vi "Charging_Configure.vi"(7 "file path (Rounded Square Wave Array)":path=path "C:/ATS Development/Code/Drivers/Charging/Rounded_Square_Wave_Array", 8 "error in (no error)":errorcluster, 10 "waveform settings":T1={"Frequency (40000 Hz)"=40000.0, "Offset (0 V)"=0.0, "Gain (3.7)"=3.7}, 11 "logical name (\"SampleFGen\")":refnum<k15> caption="instrument handle") -> (0 "error out":errorcluster, 1 "Arbitrary Waveform Handle [ARB]":i32, 3 "instrument handle out":refnum<k15>)   [LabVIEW 2010]
uses:
  <vilib>/Utility/file.llb/Read From Spreadsheet File (DBL).vi
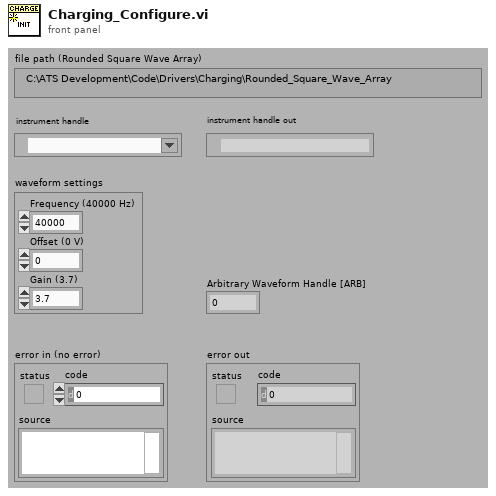
[diagram p1: front panel]
types:
  T1 = cluster{"Frequency (40000 Hz)":dbl, "Offset (0 V)":dbl, "Gain (3.7)":dbl}
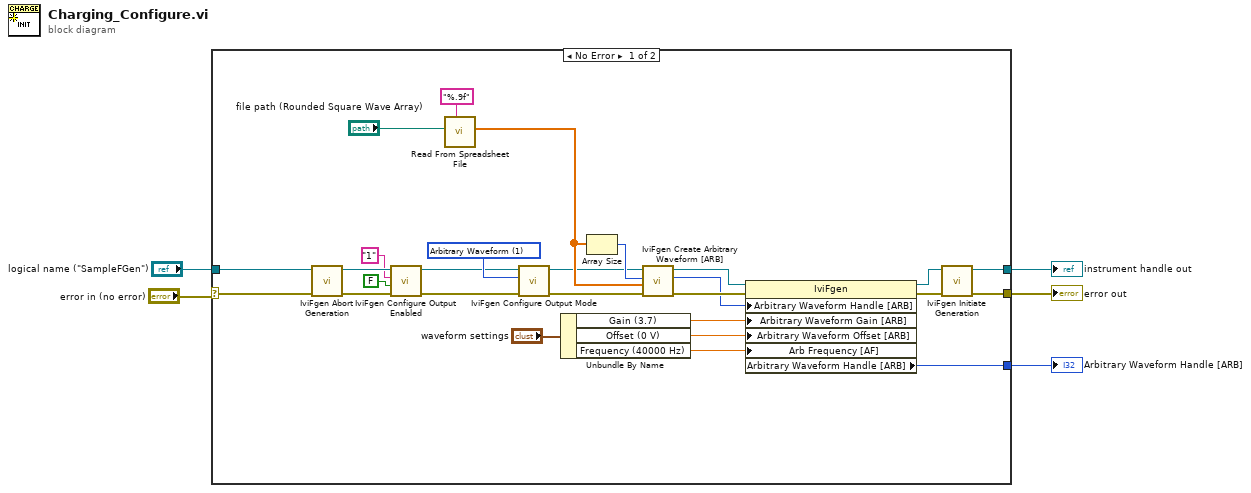
[diagram p0: block diagram]
diagram:
  n1 = case shown="No Error" "error in (no error)" {
    selector: "error in (no error)" -> [w30 w34]
    tunnel: [w6 w34] -> w4
    tunnel: "logical name (\"SampleFGen\")" -> [w16 w33]
    tunnel: [w21 _] -> w1
    tunnel: [w7 w33] -> w2
    frame No Error {
      w29 = 1 items=["Standard Function", "Arbitrary Waveform", "Arbitrary Sequence"] ("output mode (Standard Function)")
      n2 = call <vilib>:"IviFgen Abort Generation.vi"("error in (no error)"=w30, "instrument handle"=w16) -> ("error out"=w9:errorcluster, "instrument handle out"=w10:refnum<k15>)  [unwired: 8 in]
      n3 = call <vilib>:"IviFgen Configure Output Enabled.vi"("error in (no error)"=w9, "channel enabled (True)"=FALSE, "channel name (\"CHANNEL1\")"="1" ("channel name (\"CHANNEL1\")"), "instrument handle"=w10) -> ("error out"=w15:errorcluster, "instrument handle out"=w14:refnum<k15>)  [unwired: 6 in]
      n4 = call-poly <vilib>:"Read From Spreadsheet File.vi"("format (%.3f)"="%.9f", "file path (dialog if empty)"="file path (Rounded Square Wave Array)") -> ("first row"=w27:dbl[])  [unwired: 5 in, 4 out]
      n5 = call <vilib>:"IviFgen Configure Output Mode.vi"("error in (no error)"=w15, "output mode (Standard Function)"=w29, "instrument handle"=w14) -> ("error out"=w11:errorcluster, "instrument handle out"=w12:refnum<k15>)  [unwired: 7 in]
      n6 = Unbundle By Name("waveform settings") -> ("Gain (3.7)"=w18:dbl, "Offset (0 V)"=w19:dbl, "Frequency (40000 Hz)"=w20:dbl)
      n7 = Array Size(array=w27) -> (size(s)=w28:i32)
      n8 = call <vilib>:"IviFgen Create Arbitrary Waveform [ARB].vi"("error in (no error)"=w11, "waveform data array (empty)"=w27, "waveform size (0)"=w28, "instrument handle"=w12) -> ("error out"=w24:errorcluster, "waveform handle"=w22:i32, "instrument handle out"=w25:refnum<k15>)  [unwired: 5 in]
      n9 = property class="IviFgen"(reference=w25, error in=w24, "Arbitrary Waveform Handle [ARB]"=w22, "Arbitrary Waveform Gain [ARB]"=w18, "Arbitrary Waveform Offset [ARB]"=w19, "Arb Frequency [AF]"=w20) -> (reference out=w26:refnum<k15>, error out=w23:errorcluster, "Arbitrary Waveform Handle [ARB]"=w21:i32)
      n10 = call <vilib>:"IviFgen Initiate Generation.vi"("error in (no error)"=w23, "instrument handle"=w26) -> ("error out"=w6:errorcluster, "instrument handle out"=w7:refnum<k15>)  [unwired: 8 in]
    }
    frame Error {
    }
  }
  "error out" <- w4
  "instrument handle out" <- w2
  "Arbitrary Waveform Handle [ARB]" <- w1
